vi "ROI grp-Event Case-Shortcut menu activ.vi"(9 "Coords":T1, 11 "[Groups] menu ref":refnum<k9>) -> (0 "error out":errorcluster)   [LabVIEW 2020]
uses:
  <vilib>/Utility/miscctls.llb/LVPoint32TypeDef.ctl
  Globals/gl_ROI grp window globals.vi
panel:
  out "menu reference out":refnum<k9>
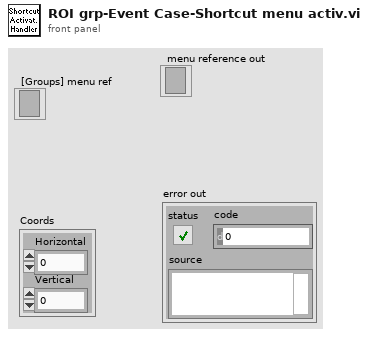
[diagram p1: front panel]
types:
  T1 = typedef "LVPoint32TypeDef.ctl" = cluster{"Horizontal":i32, "Vertical":i32}
  T2 = typedef "ROI grp-window ctrl refs.ctl" = cluster{"This VI":refnum<vi>, "Pane":refnum<vi>, "Table":refnum<vi>}
  T3 = typedef "LVRowAndColumnTypeDef.ctl" = cluster{"Row":i32, "Column":i32}
  T4 = cluster{"Valid row selected?":bool, "Valid column selected?":bool}
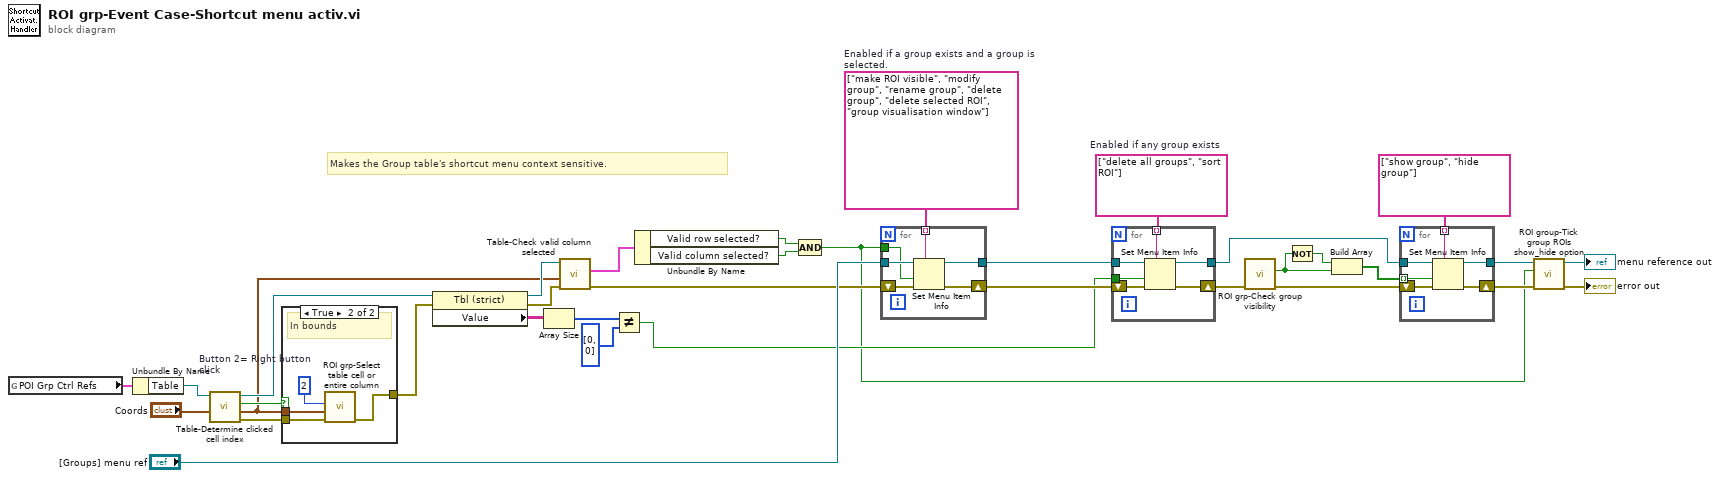
[diagram p0: block diagram]
diagram:
  w34 = string[] ["delete all groups", "sort ROI"]  # Enabled if any group exists
  w35 = string[] ["make ROI visible", "modify group", "rename group", "delete group", "delete selected ROI", "group visualisation window"]  # Enabled if a group exists and a group is selected.
  # "Makes the Group table's shortcut menu context sensitive."
  n1 = global read "gl_ROI grp window globals.vi" "POI Grp Ctrl Refs"() -> (w30:T2)
  n2 = Unbundle By Name(w30) -> ("Table"=w16:refnum<vi>)
  n3 = call <userlib>:"Table-Determine clicked cell index.vi"("Coords"="Coords", "Table in"=w16) -> ("error out"=w21:errorcluster, "Cell Position"=w13:T3, "In Bounds?"=w22:bool, "Table out"=w15:refnum<vi>)  [unwired: 6 in]
  n4 = case shown="True" w22 {
    tunnel: w13 -> [_ w40]
    tunnel: w21 -> [w36 w39]
    tunnel: [w36 w38] -> w20
    frame False {
    }
    frame True {
      w37 = u16 2  # Button 2= Right button click
      # "In bounds"
      n5 = call "ROI grp-Select table cell or entire column.vi"("error in (no error)"=w39, "Cell Position"=w40, "Button (1=left 2=right)"=w37) -> ("error out"=w38:errorcluster)  [unwired: 8 in]
    }
  }
  n6 = property class="Tbl (strict)"(reference=w15, error in=w20) -> (reference out=w26:refnum<vi>, error out=w25:errorcluster, "Value"=w29:string[][])
  n7 = Array Size(array=w29) -> (size(s)=w28:i32[])
  n8 = call <userlib>:"Table-Check valid column selected.vi"("error in (no error)"=w25, "Cell Position"=w13, "Table ref in"=w26) -> ("error out"=w24:errorcluster, "Selected cell validity cluster"=w17:T4)  [unwired: 4 in, 3 out]
  n9 = Not Equal?(x=w28, y=i32[] [0, 0]) -> (x != y?=w23:bool)
  n10 = Unbundle By Name(w17) -> ("Valid row selected?"=w19:bool, "Valid column selected?"=w18:bool)
  n11 = Compound Arithmetic op=AND(w19, w18) -> (w1:bool)
  n12 = for {
    tunnel: "[Groups] menu ref" -> [w46]
    tunnel: w35 -> [w45] mode=indexing
    tunnel: w1 -> [w44]
    tunnel: [w43] -> w33
    shift-right: [w41] -> w32
    shift-left: w24 -> [w42]
    n13 = Set Menu Item Info(7:w45, 8:w42, 9:w44, 11:w46) -> (0:w41:errorcluster, 3:w43:refnum<k9>)  [unwired: 3 in]
  }
  n14 = for {
    tunnel: w33 -> [w52]
    tunnel: w34 -> [w51] mode=indexing
    tunnel: w23 -> [w50]
    shift-right: [w48] -> w11
    shift-left: w32 -> [w49]
    tunnel: [w47] -> w12
    n15 = Set Menu Item Info(7:w51, 8:w49, 9:w50, 11:w52) -> (0:w48:errorcluster, 3:w47:refnum<k9>)  [unwired: 3 in]
  }
  n16 = call "ROI grp-Check group visibility.vi"("error in (no error)"=w11) -> ("error out"=w10:errorcluster, "Group is visible"=w7:bool)  [unwired: 9 in]
  n17 = Not(x=w7) -> (.not. x?=w8:bool)
  n18 = Build Array(w8, w7) -> (w6:bool[])
  n19 = for {
    tunnel: w12 -> [w58]
    tunnel: string[] ["show group", "hide group"] -> [w57] mode=indexing
    tunnel: w6 -> [w54] mode=indexing
    shift-right: [w55] -> w5
    shift-left: w10 -> [w56]
    tunnel: [w53] -> w4
    n20 = Set Menu Item Info(7:w57, 8:w56, 9:w54, 11:w58) -> (0:w55:errorcluster, 3:w53:refnum<k9>)  [unwired: 3 in]
  }
  n21 = call "ROI group-Tick group ROIs show_hide option.vi"("error in (no error)"=w5, "Valid?"=w1, "Menu in"=w4) -> ("error out"=→"error out":errorcluster, "Menu out"=→"menu reference out":refnum<k9>)  [unwired: 7 in]
